vi "New Execution.vi"(8 "error in (no error)":errorcluster, 11 "Execution Options (Default)":T1={"Use Default Model (T)"=TRUE, "Release Related References (T)"=TRUE}) -> (0 "error out":errorcluster, 3 "Execution out":refnum<class "Execution.lvclass">)   [LabVIEW 2020, in "TSnax.lvlib" / "Execution.lvclass"]
uses:
  Execution.lvclass
  Execution Options.ctl
  Execution.lvclass/Execution.ctl
  Engine/Engine.lvclass
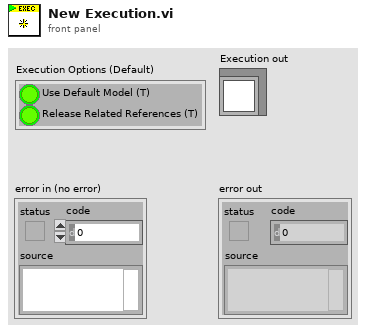
[diagram p1: front panel]
types:
  T1 = typedef "TSnax.lvlib/Execution.lvclass/Execution Options.ctl" = cluster{"Use Default Model (T)":bool, "Release Related References (T)":bool}
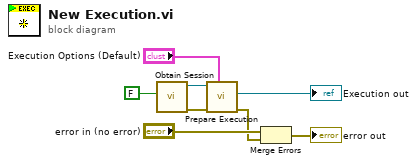
[diagram p0: block diagram]
diagram:
  n1 = call "Obtain Session.vi"("Create if needed? (T)"=FALSE) -> ("error out"=w7:errorcluster, "Engine out"=w6:refnum<class "Engine.lvclass">)  [unwired: 9 in]
  n2 = call "Prepare Execution.vi"("Options (Default)"="Execution Options (Default)", "error in (no error)"=w7, "Engine in"=w6) -> ("error out"=w2:errorcluster, "Execution"=→"Execution out":refnum<class "Execution.lvclass">)  [unwired: 6 in, 1 out]
  n3 = Merge Errors("error in (no error)", w2) -> (→"error out":errorcluster)
